vi "ExSubTTLnDACoutput.vi"(2 "error in (no error)":errorcluster, 3 "Value to Output":u32, 4 "Port":u32, 5 "Camera Handle":u32) -> (0 "error out":errorcluster, 1 "Camera Handle":u32)   [LabVIEW 2010]
panel:
  # "ExSubTTLnDACoutput.vi : this sub-vi sets the Cascade TTL lines and\n2 DAC lines. by setting the port determines which is used.\nSee page 37 and 38 in Cascade manual for more information."
  # "For cascade this value can be 0-5\n0-3 is TTL\n4-5 is DAC"
  # "For DAC's this value can be 0-255, for Cascade TTL this value can be 0-3"
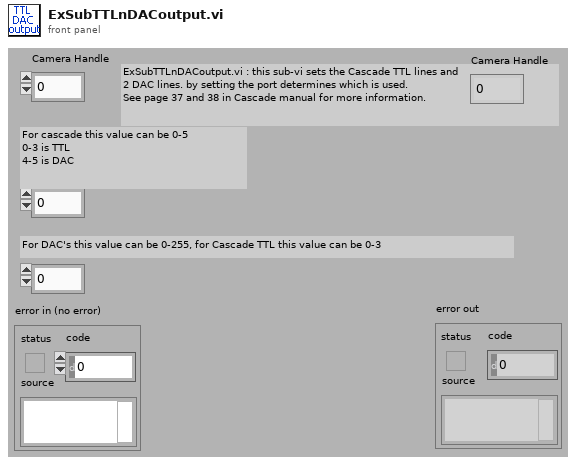
[diagram p1: front panel]
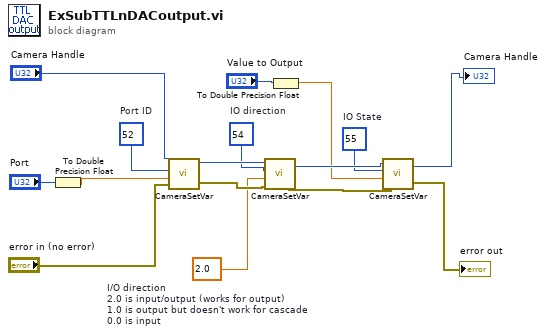
[diagram p0: block diagram]
diagram:
  w5 = 55  # IO State
  w8 = 2.0  # I/O direction 2.0 is input/output (works for output) 1.0 is output but doesn't work for cascade 0.0 is input
  w9 = 54  # IO direction
  w16 = 52  # Port ID
  n1 = To Double Precision Float(number="Port") -> (double precision float=w13:dbl)
  n2 = call <userlib>:"CameraSetVar.vi"("error in"="error in (no error)", "Value"=w13, "Parameter ID"=w16, "Camera Handle"="Camera Handle") -> ("error out"=w11:errorcluster, "CameraHandle"=w10:u32)
  n3 = call <userlib>:"CameraSetVar.vi"("error in"=w11, "Value"=w8, "Parameter ID"=w9, "Camera Handle"=w10) -> ("error out"=w7:errorcluster, "CameraHandle"=w6:u32)
  n4 = To Double Precision Float(number="Value to Output") -> (double precision float=w3:dbl)
  n5 = call <userlib>:"CameraSetVar.vi"("error in"=w7, "Value"=w3, "Parameter ID"=w5, "Camera Handle"=w6) -> ("error out"=→"error out":errorcluster, "CameraHandle"=→"Camera Handle":u32)
